vi "Write_frames.vi"(8 "error in (no error)":errorcluster, 9 "Channel":u16, 10 "CAN_MSGs_Write":T1 {"CAN_Frames"."Payload" format="%.0x"; "CAN_Frames"."MSGTYPE" items=["STATUS"=128, "EXTENDED"=2, "RTR"=1, "DATA MSG"=0]; "CAN_Frames"."CAN_ID" format="%.0x"}, 11 "DLL_Path":path) -> (0 "error out":errorcluster, 3 "CAN_bit frame":bool[][](array[boolean]))   [LabVIEW 2024, in "PCANusb_DTU.lvlib"]
uses:
  PCANusb_DTU.lvlib
  CAN_MSGs.ctl
  CAN_Frames_ctrl.ctl
  Framing datas.ctl
  PCAN_Global.vi
  <userlib>/PCANBasic/PCANBasic.lvlib
  c7c5d167-9c6a-4621-beea-81a398c89069.vi
panel:
  out "function return":u32 format="%.0x"
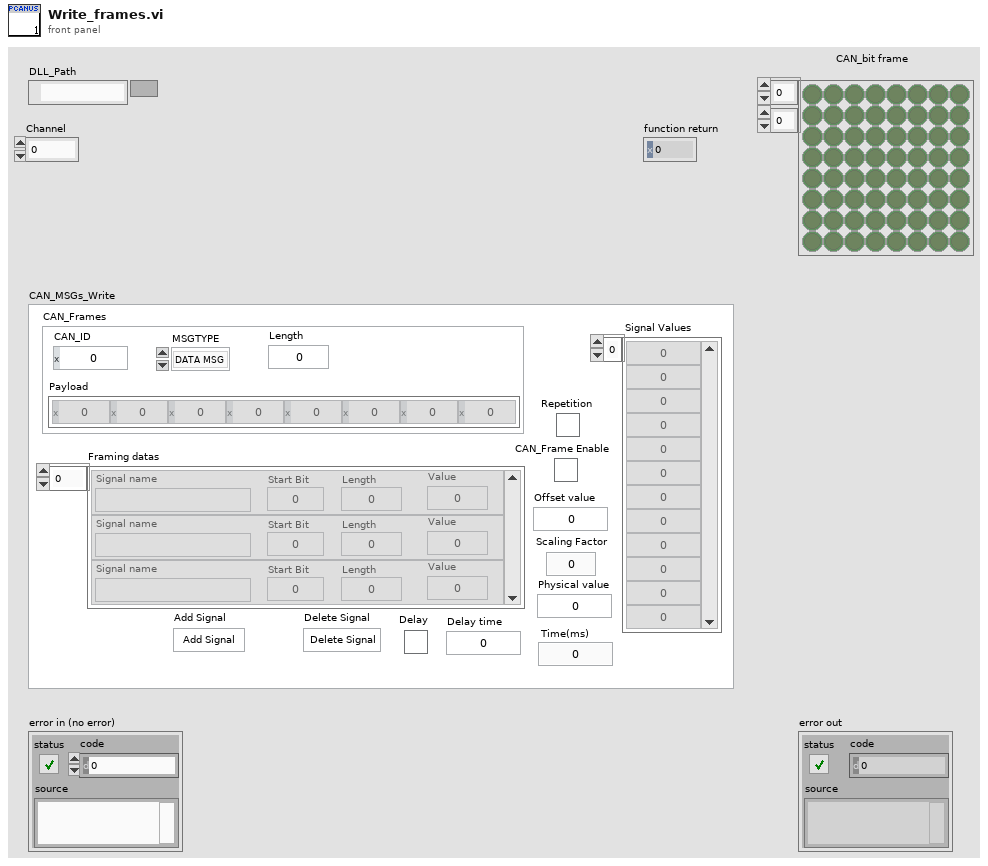
[diagram p1: front panel]
types:
  T1 = typedef "PCANusb_DTU.lvlib/CAN_MSGs.ctl" = cluster{"Scaling Factor":u16, "Physical value":dbl, "CAN_Frames":T2, "Offset value":dbl, "Framing datas":T3[], "CAN_Frame Enable":bool, "Add Signal":bool, "Delete Signal":bool, "Signal Values":dbl[], "Time(ms)":dbl, "Repetition":bool, "Delay":bool, "Delay time":dbl}
  T2 = typedef "PCANusb_DTU.lvlib/CAN_Frames_ctrl.ctl" = cluster{"CAN_ID":u32, "MSGTYPE":u8, "Payload":u8[], "Length":u8}
  T3 = typedef "PCANusb_DTU.lvlib/Framing datas.ctl" = cluster{"Signal name":string, "Start Bit":u8, "Length":u8, "Value":u16}
  T4 = cluster{"ID":u32, "MSGTYPE":u8, "LEN":u8, "DATA[0]":u8, "DATA[1]":u8, "DATA[2]":u8, "DATA[3]":u8, "DATA[4]":u8, "DATA[5]":u8, "DATA[6]":u8, "DATA[7]":u8}
  T5 = cluster{"ID":u32, "MSGTYPE":u8, "LEN":u8, "Data":u8[]}
  T6 = typedef "PCANusb.lvlib/CAN_MSGs.ctl" = cluster{"Scaling Factor":u16, "Physical value":dbl, "CAN_Frames":T7, "Offset value":dbl, "Framing datas":T8[], "CAN_Frame Enable":bool, "Add Signal":bool, "Delete Signal":bool, "Signal Values":dbl[], "Time(ms)":dbl, "Repetition":bool, "Delay":bool, "Delay time":dbl}
  T7 = typedef "PCANusb.lvlib/CAN_Frames_ctrl.ctl" = cluster{"CAN_ID":u32, "MSGTYPE":u8, "Payload":u8[], "Length":u8}
  T8 = typedef "PCANusb.lvlib/Framing datas.ctl" = cluster{"Signal name":string, "Start Bit":u8, "Length":u8, "Value":u16}
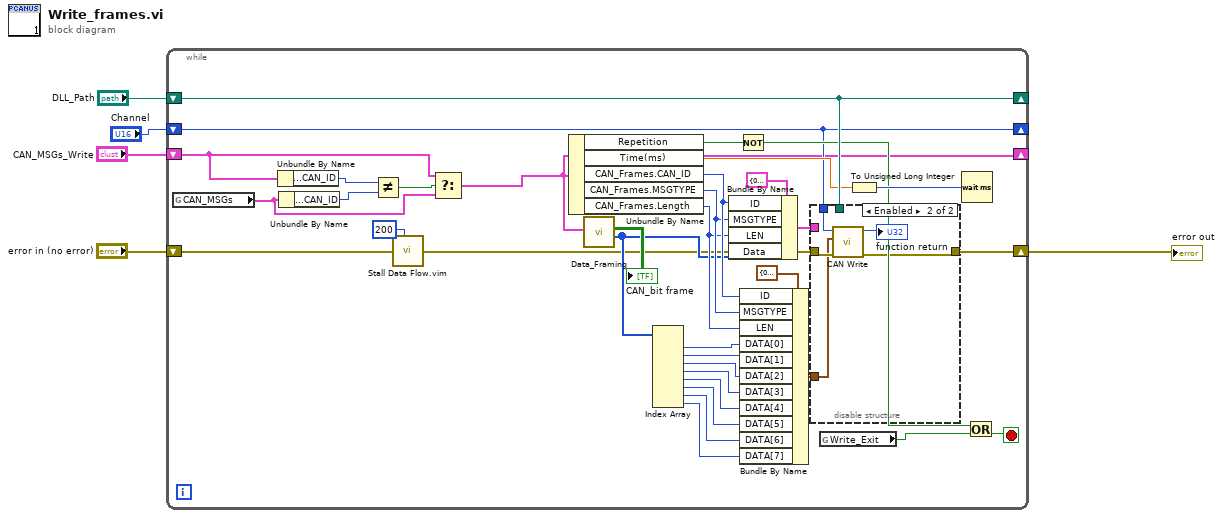
[diagram p0: block diagram]
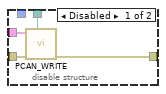
[diagram p2: hidden frame]
diagram:
  n1 = while {
    shift-right: [w40] -> w5
    shift-left: "error in (no error)" -> [w36]
    shift-right: [w10] -> _
    shift-left: "CAN_MSGs_Write" -> [w12]
    shift-right: [w35] -> _
    shift-left: "DLL_Path" -> [w35]
    shift-right: [w15] -> _
    shift-left: "Channel" -> [w15]
    stop <- w32 stop-if-true
    n2 = global read "PCAN_Global.vi" "CAN_MSGs"() -> (w9:T6)
    n3 = Unbundle By Name(w12) -> ("CAN_Frames.CAN_ID"=w14:u32)
    n4 = Unbundle By Name(w9) -> ("CAN_Frames.CAN_ID"=w13:u32)
    n5 = Not Equal?(x=w14, y=w13) -> (x != y?=w11:bool)
    n6 = call "Stall Data Flow.vim"("value in"=w36, "milliseconds to wait"=u32 200) -> ("value out"=w7:errorcluster)  [unwired: 1 out]
    n7 = Select(t=w12, s=w11, f=w9) -> (s? t:f=w10:T6)
    n8 = Unbundle By Name(w10) -> ("Repetition"=w31:bool, "Time(ms)"=w34:dbl, "CAN_Frames.CAN_ID"=w28:u32, "CAN_Frames.MSGTYPE"=w27:u8, "CAN_Frames.Length"=w26:u8)
    n9 = call "Data_Framing.vi"("CAN_MSGs"=w10) -> ("CAN_data frame"=w25:u8[], "CAN_bit frame"=→"CAN_bit frame":bool[][])  [unwired: 9 in]
    n10 = Index Array(array=w25) -> (element #1=w24:u8, element #2=w23:u8, element #3=w22:u8, element #4=w21:u8, element #5=w20:u8, element #6=w19:u8, element #7=w18:u8, element #8=w17:u8)  [unwired: 8 in]
    n11 = Bundle By Name(cluster=T5 {"ID"=0, "MSGTYPE"=128, "LEN"=0, "Data"=[]} ("TPCANMsg"), "ID"=w28, "MSGTYPE"=w27, "LEN"=w26, "Data"=w25) -> (w37:T5)
    n12 = Not(x=w31) -> (.not. x?=w30:bool)
    n13 = Bundle By Name(cluster=T4 {"ID"=0, "MSGTYPE"=0, "LEN"=0, "DATA[0]"=0, "DATA[1]"=0, "DATA[2]"=0, "DATA[3]"=0, "DATA[4]"=0, "DATA[5]"=0, "DATA[6]"=0, "DATA[7]"=0} ("MessageBuffer"), "ID"=w28, "MSGTYPE"=w27, "LEN"=w26, "DATA[0]"=w24, "DATA[1]"=w23, "DATA[2]"=w22, "DATA[3]"=w21, "DATA[4]"=w20, "DATA[5]"=w19, "DATA[6]"=w18, "DATA[7]"=w17) -> (w16:T4)
    n14 = disable-structure shown="Enabled" {
      disable-tunnel: [w44 w49] -> w40
      disable-tunnel: w37 -> [w43 _]
      disable-tunnel: w7 -> [w42 w48]
      disable-tunnel: w35 -> [w41 _]
      disable-tunnel: w16 -> [_ w47]
      disable-tunnel: w15 -> [_ w46]
      frame Disabled {
        n15 = call <vilib>:"PCAN_WRITE.vi"("path in"=w41, "error in (no error)"=w42, "TPCANMsg"=w43) -> ("error out"=w44:errorcluster)  [unwired: 6 in, 2 out]
      }
      frame Enabled {
        n16 = call <userlib>:"CAN Write.vi"("error in (no error)"=w48, "MessageBuffer"=w47, "Channel"=w46) -> ("error out"=w49:errorcluster, "function return"=→"function return":u32)  [unwired: 6 in, 1 out]
      }
    }
    n17 = global read "PCAN_Global.vi" "Write_Exit"() -> (w8:bool)
    n18 = To Unsigned Long Integer(number=w34) -> (unsigned 32bit integer=w33:u32)
    n19 = Wait (ms)(milliseconds to wait=w33) -> ()  [unwired: 1 out]
    n20 = Or(x=w30, y=w8) -> (x .or. y?=w32:bool)
  }
  "error out" <- w5
